vi "SetHardConf.vi"(7 "Params Values":T1(array[cluster]), 8 "error in (no error)":errorcluster, 10 "Channel":u8, 11 "ID In":i32) -> (0 "error out":errorcluster, 2 "Params Values Trimed":T1(array[cluster]), 3 "ID Out":i32)   [LabVIEW 2022 SP3, in "EClib functions.lvlib"]
doc: "This VI sets the hardware configuration on the selected channel.\nUsed to set the connection type (EC_TO_GROUND) for VMP4 series"
uses:
  EClib functions.lvlib
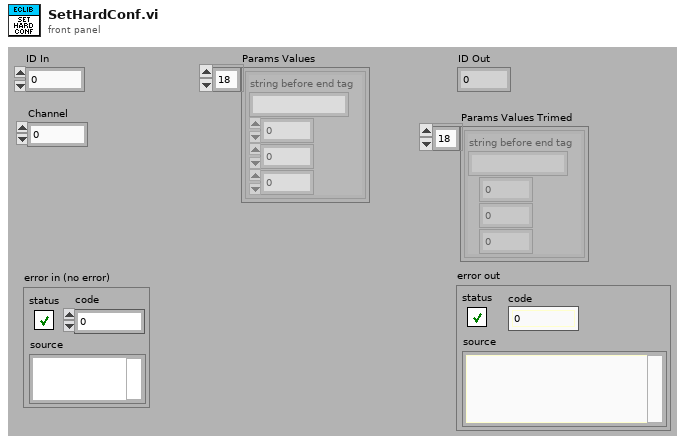
[diagram p1: front panel]
types:
  T1 = cluster{"string before end tag":string, i32, i32, i32}[]
  T2 = enum16{"unknown", "essential", "premium", "premium digicore"}
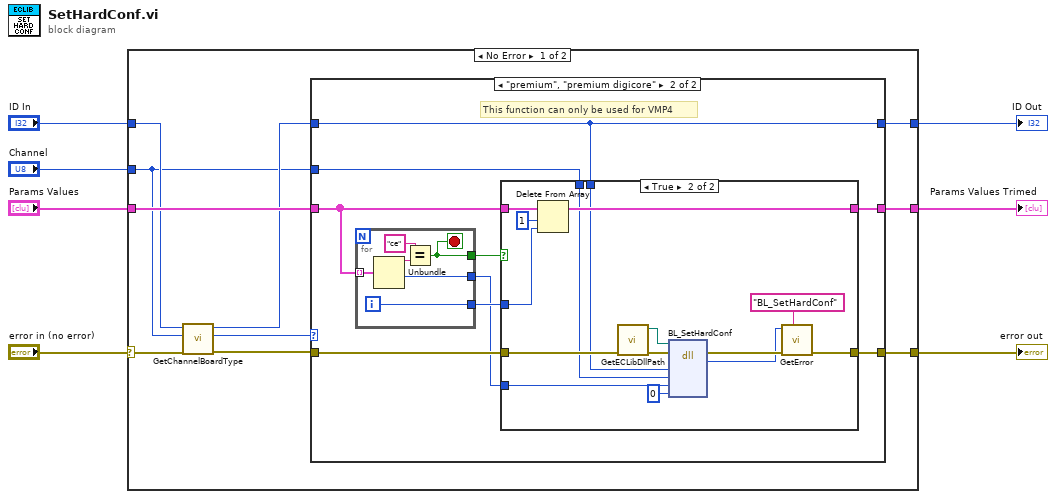
[diagram p0: block diagram]
diagram:
  n1 = case shown="No Error" "error in (no error)" {
    selector: "error in (no error)" -> [w12 w55]
    tunnel: [w17 w55] -> w1
    tunnel: "ID In" -> [w9 w54]
    tunnel: "Channel" -> [w8 _]
    tunnel: [w14 w54] -> w5
    tunnel: "Params Values" -> [w16 w53]
    tunnel: [w15 w53] -> w3
    frame No Error {
      n2 = call "GetChannelBoardType.vi"("error in (no error)"=w12, "Channel"=w8, "ConnectionID IN"=w9) -> ("error out"=w11:errorcluster, "BoardType"=w13:T2, "ConnectionID Out"=w10:i32)  [unwired: 5 in, 1 out]
      n3 = case shown="\"premium\", \"premium digicore\"" w13 {
        tunnel: w8 -> [_ w29]
        tunnel: w11 -> [w19 w28]
        tunnel: w10 -> [w18 w21]
        tunnel: [w19 w27] -> w17
        tunnel: w16 -> [w20 w24]
        tunnel: [w20 w23] -> w15
        tunnel: [w18 w21] -> w14
        frame "unknown", "essential" {
        }
        frame "premium", "premium digicore" {
          # "This function can only be used for VMP4"
          n4 = for {
            tunnel: w24 -> [w52] mode=indexing
            tunnel: [w49] -> w26
            tunnel: [w48] -> w22
            tunnel: [w47] -> w25
            i -> [w49]
            stop <- w48 stop-if-true
            n5 = Unbundle(w52) -> ("string before end tag"=w51:string, w47:i32)  [unwired: 2 out]
            n6 = Equal?(x="ce", y=w51) -> (x = y?=w48:bool)
          }
          n7 = case shown="True" w22 {
            tunnel: w29 -> [_ w35]
            tunnel: w28 -> [w30 w46]
            tunnel: w21 -> [_ w36]
            tunnel: [w30 w32] -> w27
            tunnel: w26 -> [_ w44]
            tunnel: w25 -> [_ w34]
            tunnel: w24 -> [w31 w43]
            tunnel: [w31 w42] -> w23
            frame False {
            }
            frame True {
              n8 = Delete From Array(array=w43, length=1, index=w44) -> (array with subset deleted=w42:T1)  [unwired: 1 out]
              n9 = call "GetECLibDllPath.vi"("error in (no error)"=w46) -> ("error out"=w41:errorcluster, "ECLibDLLPath"=w37:path)  [unwired: 9 in]
              n10 = dll-call lib="?" fn="BL_SetHardConf"(path in=w37, error in=w41, "arg1"=w36, "arg2"=w35, "Conn"=w34, "Ground"=0) -> (error out=w40:errorcluster, "return type"=w38:i32)  [unwired: 5 in, 1 out]
              n11 = call "GetError.vi"("DLLFunction"="BL_SetHardConf", "error in"=w40, "code"=w38) -> ("error out"=w32:errorcluster)  [unwired: 8 in]
            }
          }
        }
      }
    }
    frame Error {
    }
  }
  "error out" <- w1
  "ID Out" <- w5
  "Params Values Trimed" <- w3
